vi "Set PIDS loop 1_MFP3D_Lucy.vi"(10 "Y Setpoint":dbl format="%#_6p") -> ()   [LabVIEW 2019]
panel:
  out "error out":errorcluster
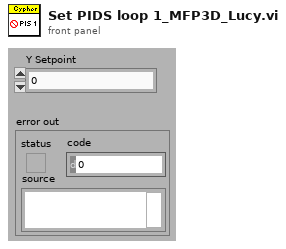
[diagram p1: front panel]
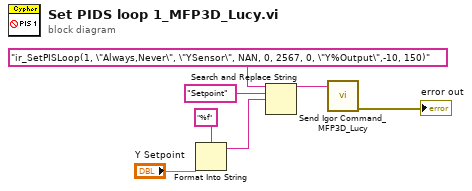
[diagram p0: block diagram]
diagram:
  n1 = Format Into String(format string="%f", "Y Setpoint") -> (resulting string=w4:string)  [unwired: 2 in, 1 out]
  n2 = Search and Replace String(input string="ir_SetPISLoop(1, \"Always,Never\", \"YSensor\", NAN, 0, 2567, 0, \"Y%Output\",-10, 150)", search string="Setpoint", replace string=w4) -> (result string=w2:string)  [unwired: 1 in, 7 out]
  n3 = call "Send Igor Command_MFP3D_Lucy.vi"("Command"=w2) -> ("error out"=→"error out":errorcluster)  [unwired: 7 in, 2 out]
